vi "Configure.vi"(8 "error in (no error)":errorcluster, 11 "Camera_Prime95B in":refnum<class "Camera_Prime95B.lvclass">) -> (0 "error out":errorcluster, 3 "Camera_Prime95B out":refnum<class "Camera_Prime95B.lvclass">)   [LabVIEW 2020, in "Camera_Prime95B.lvlib" / "Camera_Prime95B.lvclass"]
uses:
  Camera_Prime95B.lvclass
  Camera New Frame Arrived Callback.vi
  Camera Status Callback.vi
  Hardware Abstraction Layer/Component/Camera/Camera/Camera.lvclass
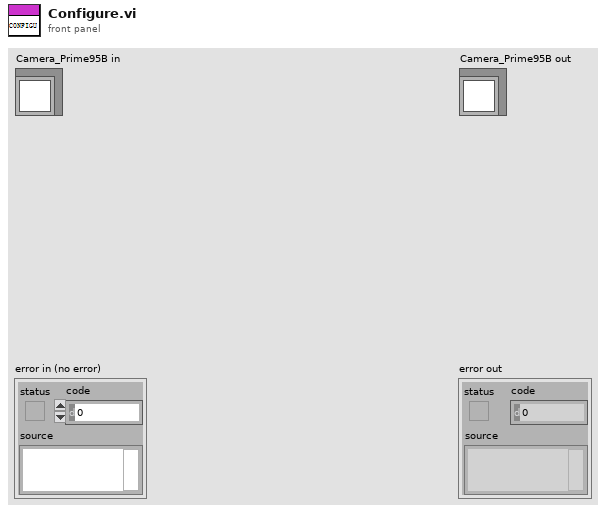
[diagram p1: front panel]
types:
  T1 = typedef "Image Type" = u32
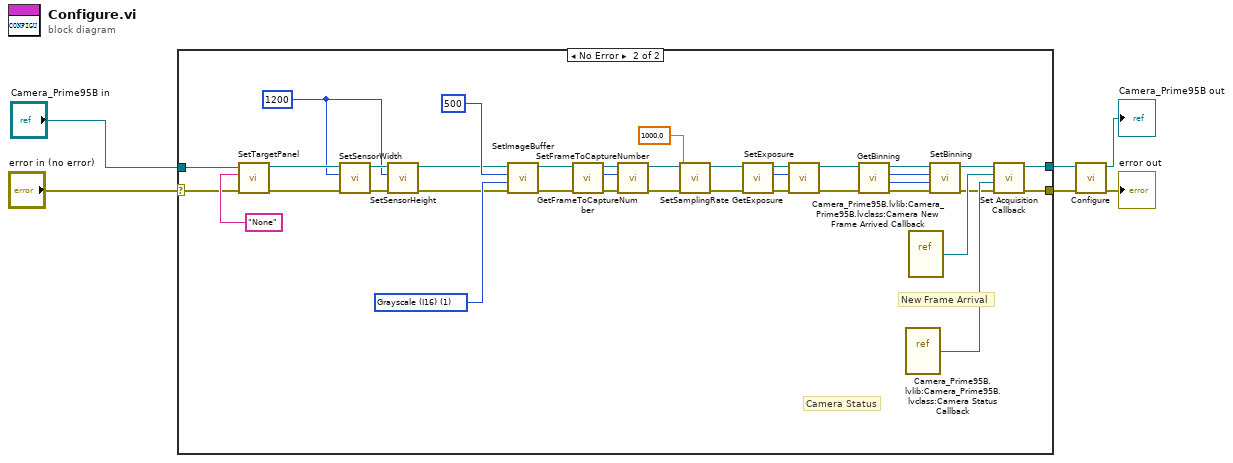
[diagram p0: block diagram]
diagram:
  n1 = case shown="No Error" "error in (no error)" {
    selector: "error in (no error)" -> [w8 w43]
    tunnel: [w8 w40] -> w3
    tunnel: "Camera_Prime95B in" -> [w7 w45]
    tunnel: [w7 w39] -> w1
    frame Error {
    }
    frame No Error {
      w13 = 1200 ("Sensor.SensorWidth(Pixel)")
      w31 = T1 1 items=["Grayscale (U8)", "Grayscale (I16)", "Grayscale (SGL)", "Complex (CSG)", "RGB (U32)", "HSL (U32)", "RGB (U64)", "Grayscale (U16)"] ("Image Type")
      # "Camera Status"
      # "New Frame Arrival"
      n2 = call-dynamic "SetTargetPanel.vi"("error in (no error)"=w43, "TargetPanel"="None" ("Sub Panel"), "GRMActor in"=w45) -> ("error out"=w42:errorcluster, "GRMActor out"=w17:refnum<class "Camera_Prime95B.lvclass">)  [unwired: 7 in]
      n3 = call-dynamic "SetSensorWidth.vi"("error in (no error)"=w42, "Sensor.SensorWidth(Pixel)"=w13, "Camera in"=w17) -> ("error out"=w18:errorcluster, "Camera out"=w15:refnum<class "Camera_Prime95B.lvclass">)  [unwired: 7 in]
      n4 = call-dynamic "SetSensorHeight.vi"("error in (no error)"=w18, "Sensor.SensorHeight(Pixel)"=w13, "Camera in"=w15) -> ("error out"=w16:errorcluster, "Camera out"=w14:refnum<class "Camera_Prime95B.lvclass">)  [unwired: 7 in]
      n5 = call-dynamic "SetImageBuffer.vi"("error in (no error)"=w16, "Image Type"=w31, "max queue size (-1, unlimited)"=500, "Camera_Prime95B in"=w14) -> ("error out"=w41:errorcluster, "Camera_Prime95B out"=w29:refnum<class "Camera_Prime95B.lvclass">)  [unwired: 6 in]
      n6 = call-dynamic "GetFrameToCaptureNumber.vi"("error in (no error)"=w41, "Camera in"=w29) -> ("error out"=w30:errorcluster, "Setting.FramesToCapture"=w27:i32, "Camera out"=w28:refnum<class "Camera_Prime95B.lvclass">)  [unwired: 7 in]
      n7 = call-dynamic "SetFrameToCaptureNumber.vi"("error in (no error)"=w30, "Setting.FramesToCapture"=w27, "Camera_Prime95B in"=w28) -> ("error out"=w33:errorcluster, "Camera_Prime95B out"=w11:refnum<class "Camera_Prime95B.lvclass">)  [unwired: 7 in]
      n8 = call-dynamic "SetSamplingRate.vi"("error in (no error)"=w33, "SamplingRate(Hz)"=1000.0, "Device in"=w11) -> ("error out"=w12:errorcluster, "Device out"=w10:refnum<class "Camera_Prime95B.lvclass">)  [unwired: 7 in]
      n9 = call-dynamic "GetExposure.vi"("error in (no error)"=w12, "Camera in"=w10) -> ("error out"=w26:errorcluster, "Setting.Exposure"=w24:i32, "Camera out"=w25:refnum<class "Camera_Prime95B.lvclass">)  [unwired: 7 in]
      n10 = call-dynamic "SetExposure.vi"("error in (no error)"=w26, "Setting.Exposure"=w24, "Camera_Prime95B in"=w25) -> ("error out"=w36:errorcluster, "Camera_Prime95B out"=w22:refnum<class "Camera_Prime95B.lvclass">)  [unwired: 7 in]
      n11 = call-dynamic "GetBinning.vi"("error in (no error)"=w36, "Camera in"=w22) -> ("error out"=w23:errorcluster, "Setting.Binning.BinY"=w19:i32, "Setting.Binning.BinX"=w20:i32, "Camera out"=w21:refnum<class "Camera_Prime95B.lvclass">)  [unwired: 6 in]
      n12 = vi-ref "Camera_Prime95B.lvlib:Camera_Prime95B.lvclass:Camera Status Callback.vi"() -> ("vi reference"=w37:refnum<vi>)
      n13 = vi-ref "Camera_Prime95B.lvlib:Camera_Prime95B.lvclass:Camera New Frame Arrived Callback.vi"() -> ("vi reference"=w38:refnum<vi>)
      n14 = call-dynamic "SetBinning.vi"("error in (no error)"=w23, "Setting.Binning.BinY"=w19, "Setting.Binning.BinX"=w20, "Camera_Prime95B in"=w21) -> ("error out"=w35:errorcluster, "Camera_Prime95B out"=w34:refnum<class "Camera_Prime95B.lvclass">)  [unwired: 6 in]
      n15 = call-dynamic "Set Acquisition Callback.vi"("error in (no error)"=w35, "Camera Status"=w37, "New Frame Arrival"=w38, "Camera_Prime95B in"=w34) -> ("error out"=w40:errorcluster, "Camera_Prime95B out"=w39:refnum<class "Camera_Prime95B.lvclass">)  [unwired: 6 in]
    }
  }
  n16 = call-parent "Configure.vi"("error in (no error)"=w3, "Device in"=w1) -> ("error out"=→"error out":errorcluster, "Device out"=→"Camera_Prime95B out":refnum<class "Camera_Prime95B.lvclass">)  [unwired: 8 in]
